vi "Modbus Status PC.vi"(0 "InterfaceData":T1 {"GenEast"."TotalFuel(L)" format="%.2f"; "GenEast"."FuelRate(L/H)" format="%.2f"; "GenEast"."ApparentPower(VA)" format="%.2f"; "GenEast"."BattVoltage(V)" format="%.2f"; "GenEast"."Freq(Hz)" format="%.2f"; "GenEast"."RunHours(hr)" format="%.2f"; "GenEast"."PowerFactor" format="%.2f"; "GenEast"."ReactivePower(VAR)" format="%.2f"; "GenEast"."ActivePower(W)" format="%.2f"; "GenWest"."TotalFuel(L)" format="%.2f"; "GenWest"."FuelRate(L/H)" format="%.2f"; "GenWest"."ApparentPower(VA)" format="%.2f"; "GenWest"."BattVoltage(V)" format="%.2f"; "GenWest"."Freq(Hz)" format="%.2f"; "GenWest"."RunHours(hr)" format="%.2f"; "GenWest"."PowerFactor" format="%.2f"; "GenWest"."ReactivePower(VAR)" format="%.2f"; "GenWest"."ActivePower(W)" format="%.2f"; "Converter Alarms 2" format="%016b"; "Converter Faults 2" format="%016b"; "Controller Faults" format="%016b"; "System Status" format="%016b"; "Converter Alarms 1" format="%016b"; "Converter Faults 1" format="%016b"; "Solar Faults" format="%016b"; "ES Rack 10 Alarms" format="%016b"; "ES Rack 9 Alarms" format="%016b"; "ES Rack 8 Alarms" format="%016b"; "ES Rack 7 Alarms" format="%016b"; "ES Rack 6 Alarms" format="%016b"; "ES Rack 5 Alarms" format="%016b"; "ES Rack 4 Alarms" format="%016b"; "ES Rack 3 Alarms" format="%016b"; "ES Rack 2 Alarms" format="%016b"; "ES Rack 1 Alarms" format="%016b"; "ES System Alarms" format="%016b"; "System Faults" format="%016b"; "ES Rack 10 Faults" format="%016b"; "ES Rack 9 Faults" format="%016b"; "ES Rack 8 Faults" format="%016b"; "ES Rack 7  Faults" format="%016b"; "ES Rack 6 Faults" format="%016b"; "ES Rack 5 Faults" format="%016b"; "ES Rack 4 Faults" format="%016b"; "ES Rack 3 Faults" format="%016b"; "ES Rack 2 Faults" format="%016b"; "ES Rack 1 Faults" format="%016b"; "ES System Faults" format="%016b"}, 5 "PC Data In":T4 {"Alarms 2" format="%016b"; "Faults 2" format="%016b"; "Alarms 1" format="%016b"; "Faults 1" format="%016b"; "Contactor FB" format="%.0b"; "DC Voltage SP" format="%2.1f"; "Clear Faults SP" format="%.0b"; "Neutral Current" format="%2.1f"; "AC Current - L2" format="%2.1f"; "AC Voltage - L2" format="%2.1f"; "Temperature" format="%2.1f"; "DC Voltage" format="%2.1f"; "AC Current SP" format="%2.1f"; "AC Voltage SP" format="%2.1f"; "Frequency SP" format="%2.1f"; "AC Frequency" format="%2.1f"; "AC Current - L1" format="%2.1f"; "AC Voltage- L1" format="%2.1f"}, 9 "FPGA Data In":T3 {"SSG Active Current" format="%2.1f"; "PV Reactive Power (L1)" format="%2.1f"; "PV Reactive Power (L2)" format="%2.1f"; "PV Total Reactive Power" format="%2.1f"; "Gen Reactive Power (L1)" format="%2.1f"; "Gen Reactive Power (L2)" format="%2.1f"; "Gen Total Reactive Power" format="%2.1f"; "SSG Reactive Power (L1)" format="%2.1f"; "SSG Reactive Power (L2)" format="%2.1f"; "SSG Total Reactive Power" format="%2.1f"; "PV Total Current" format="%2.1f"; "PV Total Voltage" format="%2.1f"; "PV Active Power (L1)" format="%2.1f"; "PV Active Power (L2)" format="%2.1f"; "PV App Power (L1)" format="%2.1f"; "PV App Power (L2)" format="%2.1f"; "PV Total Active Power" format="%2.1f"; "PV Total App Power" format="%2.1f"; "PV Arms (L1)" format="%2.1f"; "PV Arms (L2)" format="%2.1f"; "PV Vrms (L1)" format="%2.1f"; "PV Vrms (L2)" format="%2.1f"; "Gen Total Current" format="%2.1f"; "SSG Total Current" format="%2.1f"; "Gen Total Voltage" format="%2.1f"; "SSG Total Voltage" format="%2.1f"; "Gen Active Power (L1)" format="%2.1f"; "Gen Active Power (L2)" format="%2.1f"; "SSG Active Power (L1)" format="%2.1f"; "SSG Active Power (L2)" format="%2.1f"; "Gen App Power (L1)" format="%2.1f"; "Gen App Power (L2)" format="%2.1f"; "SSG App Power (L1)" format="%2.1f"; "SSG App Power (L2)" format="%2.1f"; "Gen Total Active Power" format="%2.1f"; "Gen Total App Power" format="%2.1f"; "Gen Arms (L1)" format="%2.1f"; "Gen Arms (L2)" format="%2.1f"; "Gen Vrms (L1)" format="%2.1f"; "Gen Vrms (L2)" format="%2.1f"; "SSG Total Active Power" format="%2.1f"; "SSG Total App Power" format="%2.1f"; "SSG Arms (L1)" format="%2.1f"; "SSG Arms (L2)" format="%2.1f"; "SSG Vrms (L1)" format="%2.1f"; "SSG Vrms (L2)" format="%2.1f"}, 11 "Error In":errorcluster) -> (4 "InterfaceData":T1 {"GenEast"."TotalFuel(L)" format="%.2f"; "GenEast"."FuelRate(L/H)" format="%.2f"; "GenEast"."ApparentPower(VA)" format="%.2f"; "GenEast"."BattVoltage(V)" format="%.2f"; "GenEast"."Freq(Hz)" format="%.2f"; "GenEast"."RunHours(hr)" format="%.2f"; "GenEast"."PowerFactor" format="%.2f"; "GenEast"."ReactivePower(VAR)" format="%.2f"; "GenEast"."ActivePower(W)" format="%.2f"; "GenWest"."TotalFuel(L)" format="%.2f"; "GenWest"."FuelRate(L/H)" format="%.2f"; "GenWest"."ApparentPower(VA)" format="%.2f"; "GenWest"."BattVoltage(V)" format="%.2f"; "GenWest"."Freq(Hz)" format="%.2f"; "GenWest"."RunHours(hr)" format="%.2f"; "GenWest"."PowerFactor" format="%.2f"; "GenWest"."ReactivePower(VAR)" format="%.2f"; "GenWest"."ActivePower(W)" format="%.2f"; "Converter Alarms 2" format="%016b"; "Converter Faults 2" format="%016b"; "Controller Faults" format="%016b"; "System Status" format="%016b"; "Converter Alarms 1" format="%016b"; "Converter Faults 1" format="%016b"; "Solar Faults" format="%016b"; "ES Rack 10 Alarms" format="%016b"; "ES Rack 9 Alarms" format="%016b"; "ES Rack 8 Alarms" format="%016b"; "ES Rack 7 Alarms" format="%016b"; "ES Rack 6 Alarms" format="%016b"; "ES Rack 5 Alarms" format="%016b"; "ES Rack 4 Alarms" format="%016b"; "ES Rack 3 Alarms" format="%016b"; "ES Rack 2 Alarms" format="%016b"; "ES Rack 1 Alarms" format="%016b"; "ES System Alarms" format="%016b"; "System Faults" format="%016b"; "ES Rack 10 Faults" format="%016b"; "ES Rack 9 Faults" format="%016b"; "ES Rack 8 Faults" format="%016b"; "ES Rack 7  Faults" format="%016b"; "ES Rack 6 Faults" format="%016b"; "ES Rack 5 Faults" format="%016b"; "ES Rack 4 Faults" format="%016b"; "ES Rack 3 Faults" format="%016b"; "ES Rack 2 Faults" format="%016b"; "ES Rack 1 Faults" format="%016b"; "ES System Faults" format="%016b"}, 15 "Error Out":errorcluster)   [LabVIEW 2014]
uses:
  Controls/PC Data.ctl
  Controls/MicroZed Config Op Mode.ctl
  Controls/FPGA Data.ctl
  Controls/Interface Data.ctl
  Controls/Gen Data.ctl
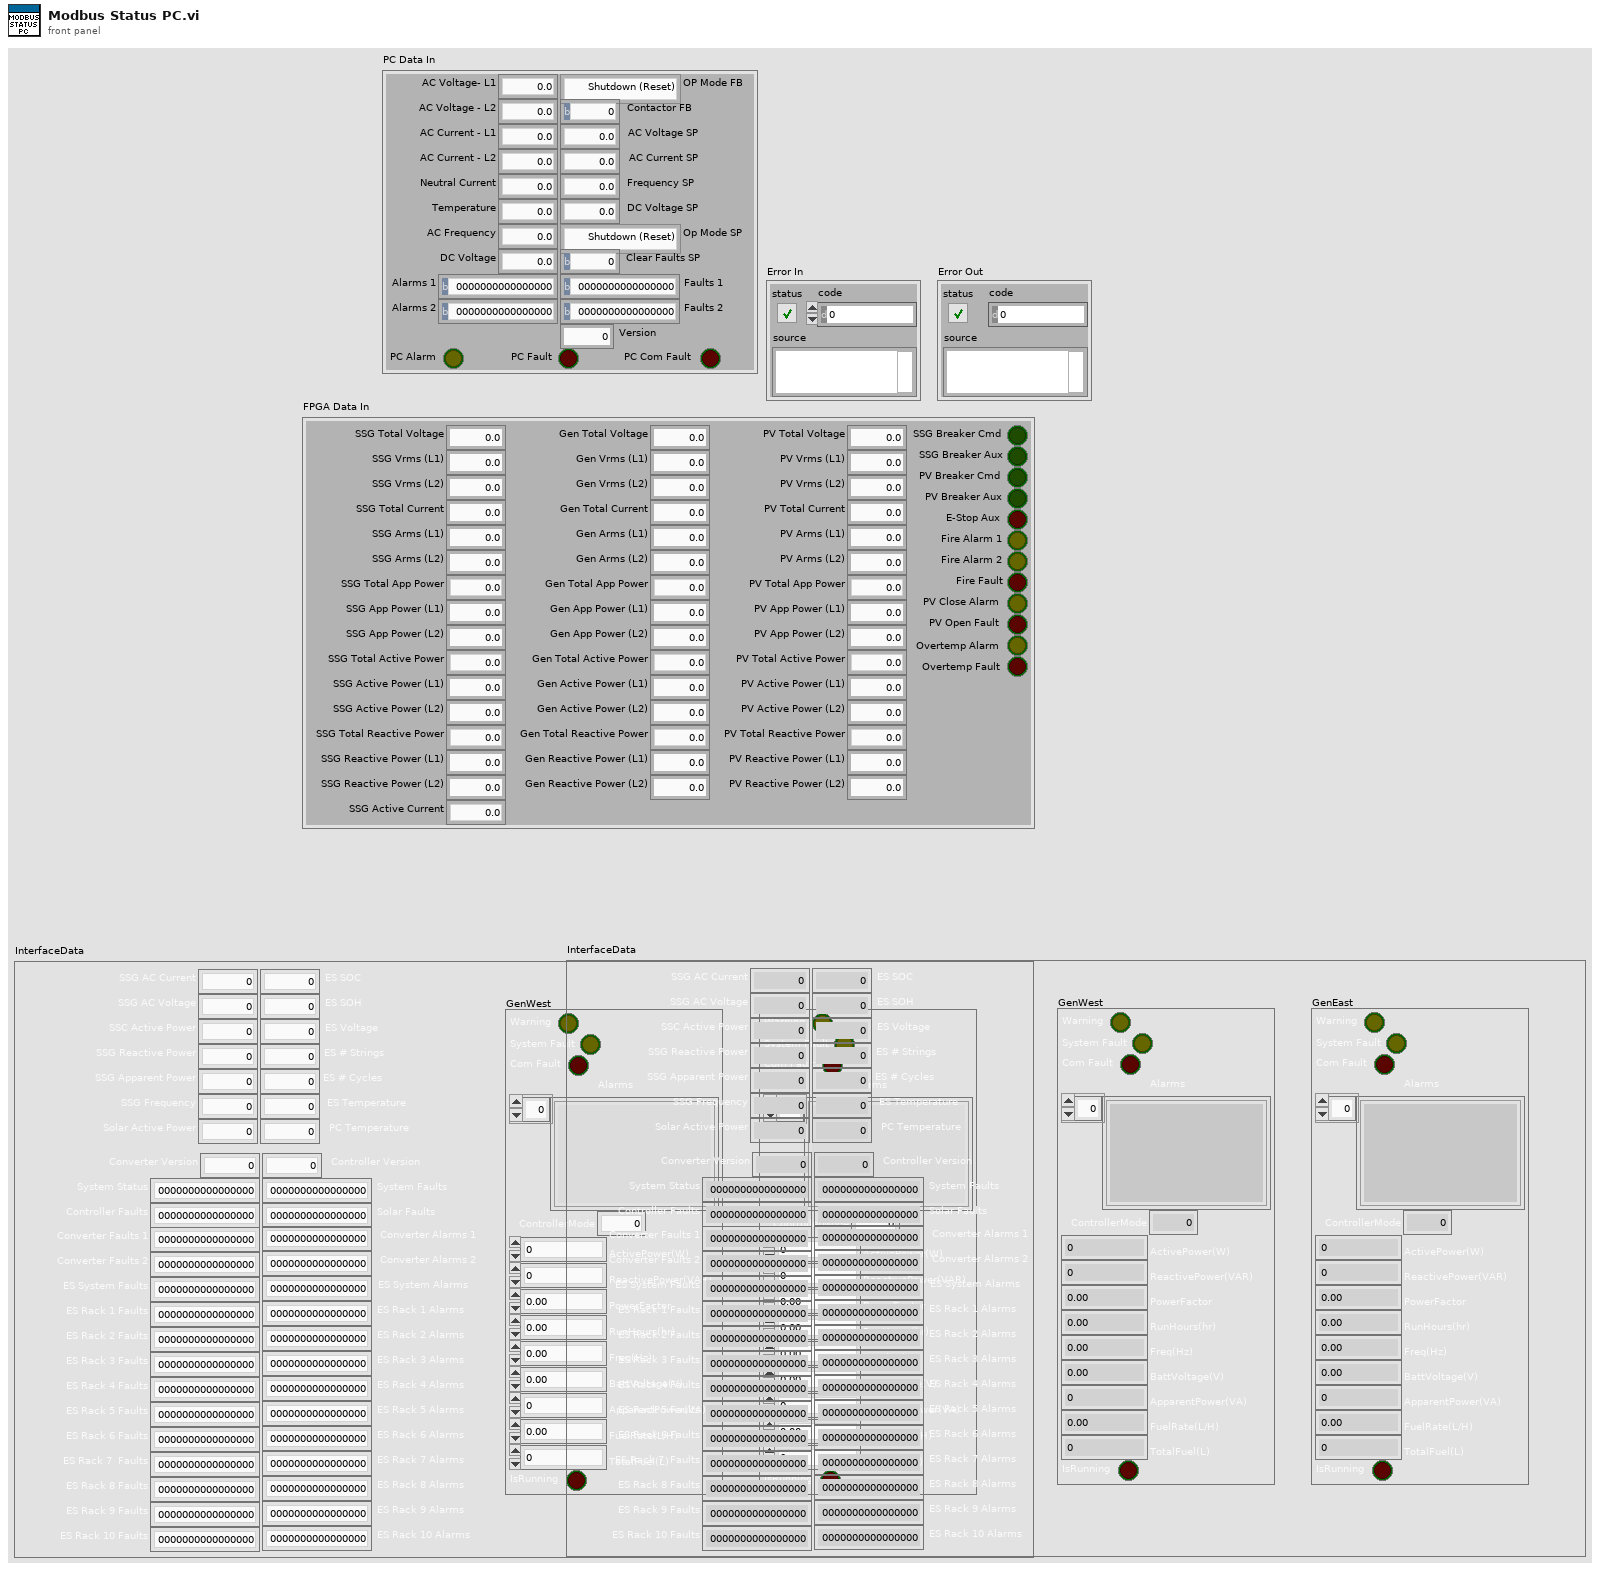
[diagram p1: front panel]
types:
  T1 = typedef "Interface Data.ctl" = cluster{"SSG AC Current":i16, "SSG AC Voltage":i16, "SSC Active Power":i16, "SSG Reactive Power":i16, "SSG Apparent Power":i16, "SSG Frequency":i16, "ES SOC":i16, "ES SOH":i16, "ES Voltage":i16, "ES # Strings":i16, "ES # Cycles":i16, "ES Temperature":i16, "PC Temperature":i16, "Solar Active Power":i16, "Converter Version":i16, "Controller Version":i16, "System Status":i16, "System Faults":i16, "Controller Faults":i16, "ES System Faults":i16, "ES System Alarms":i16, "Converter Faults 1":i16, "Converter Faults 2":i16, "Converter Alarms 1":i16, "Converter Alarms 2":i16, "Solar Faults":i16, "ES Rack 1 Faults":i16, "ES Rack 2 Faults":i16, "ES Rack 3 Faults":i16, "ES Rack 4 Faults":i16, "ES Rack 5 Faults":i16, "ES Rack 6 Faults":i16, "ES Rack 7  Faults":i16, "ES Rack 8 Faults":i16, "ES Rack 9 Faults":i16, "ES Rack 10 Faults":i16, "ES Rack 1 Alarms":i16, "ES Rack 2 Alarms":i16, "ES Rack 3 Alarms":i16, "ES Rack 4 Alarms":i16, "ES Rack 5 Alarms":i16, "ES Rack 6 Alarms":i16, "ES Rack 7 Alarms":i16, "ES Rack 8 Alarms":i16, "ES Rack 9 Alarms":i16, "ES Rack 10 Alarms":i16, "GenWest":T2, "GenEast":T2}
  T2 = typedef "Gen Data.ctl" = cluster{"Warning":bool, "System Fault":bool, "Com Fault":bool, "Alarms":string[], "ControllerMode":u16, "ActivePower(W)":i32, "ReactivePower(VAR)":i32, "PowerFactor":dbl, "RunHours(hr)":dbl, "Freq(Hz)":dbl, "BattVoltage(V)":dbl, "ApparentPower(VA)":i32, "FuelRate(L/H)":dbl, "TotalFuel(L)":u32, "IsRunning":bool}
  T3 = typedef "FPGA Data.ctl" = cluster{"Gen Total Voltage":dbl, "Gen Vrms (L1)":dbl, "Gen Vrms (L2)":dbl, "Gen Total Current":dbl, "Gen Arms (L1)":dbl, "Gen Arms (L2)":dbl, "Gen Total App Power":dbl, "Gen App Power (L1)":dbl, "Gen App Power (L2)":dbl, "Gen Total Active Power":dbl, "Gen Active Power (L1)":dbl, "Gen Active Power (L2)":dbl, "Gen Total Reactive Power":dbl, "Gen Reactive Power (L1)":dbl, "Gen Reactive Power (L2)":dbl, "SSG Total Voltage":dbl, "SSG Vrms (L1)":dbl, "SSG Vrms (L2)":dbl, "SSG Total Current":dbl, "SSG Arms (L1)":dbl, "SSG Arms (L2)":dbl, "SSG Total App Power":dbl, "SSG App Power (L1)":dbl, "SSG App Power (L2)":dbl, "SSG Total Active Power":dbl, "SSG Active Power (L1)":dbl, "SSG Active Power (L2)":dbl, "SSG Total Reactive Power":dbl, "SSG Reactive Power (L1)":dbl, "SSG Reactive Power (L2)":dbl, "PV Total Voltage":dbl, "PV Vrms (L1)":dbl, "PV Vrms (L2)":dbl, "PV Total Current":dbl, "PV Arms (L1)":dbl, "PV Arms (L2)":dbl, "PV Total App Power":dbl, "PV App Power (L1)":dbl, "PV App Power (L2)":dbl, "PV Total Active Power":dbl, "PV Active Power (L1)":dbl, "PV Active Power (L2)":dbl, "PV Total Reactive Power":dbl, "PV Reactive Power (L1)":dbl, "PV Reactive Power (L2)":dbl, "SSG Breaker Cmd":bool, "SSG Breaker Aux":bool, "PV Breaker Cmd":bool, "PV Breaker Aux":bool, "E-Stop Aux":bool, "Fire Alarm 1":bool, "Fire Alarm 2":bool, "Fire Fault":bool, "PV Close Alarm":bool, "SSG Active Current":dbl, "Overtemp Alarm":bool, "Overtemp Fault":bool, "PV Open Fault":bool}
  T4 = typedef "PC Data.ctl" = cluster{"AC Voltage- L1":dbl, "AC Voltage - L2":dbl, "AC Current - L1":dbl, "AC Current - L2":dbl, "Neutral Current":dbl, "Temperature":dbl, "AC Frequency":dbl, "DC Voltage":dbl, "AC Voltage SP":dbl, "AC Current SP":dbl, "Frequency SP":dbl, "Op Mode SP":T5, "Clear Faults SP":u16, "PC Com Fault":bool, "PC Fault":bool, "DC Voltage SP":dbl, "OP Mode FB":T5, "Contactor FB":u16, "Faults 1":u16, "Alarms 1":u16, "Faults 2":u16, "Alarms 2":u16, "PC Alarm":bool, "Version":u16}
  T5 = typedef "MicroZed Config Op Mode.ctl" = enum16{"Shutdown (Reset)", "Startup", "Idle", "Voltage Mode", "Current Mode", "Fault", "OL Voltage (Debug)", "No Data"}
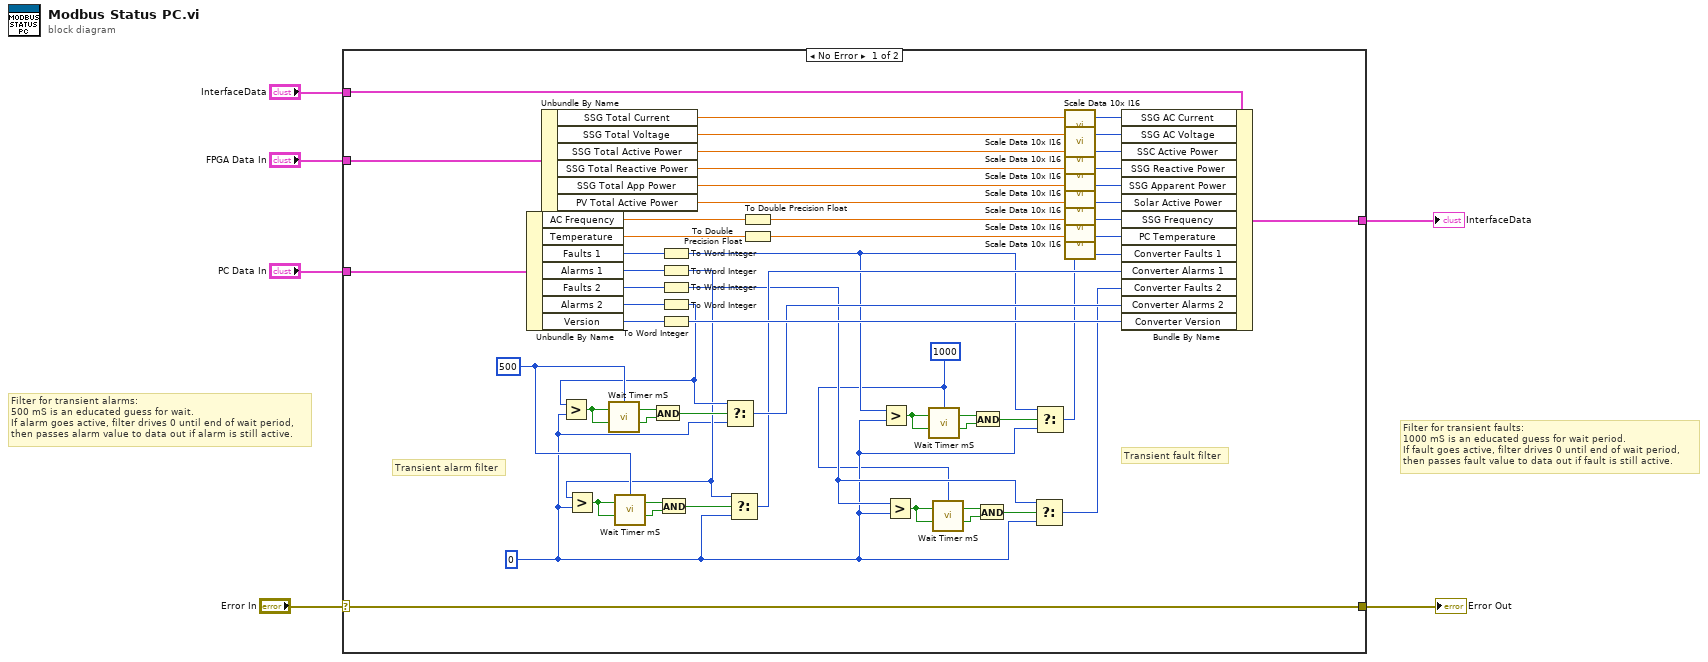
[diagram p0: block diagram]
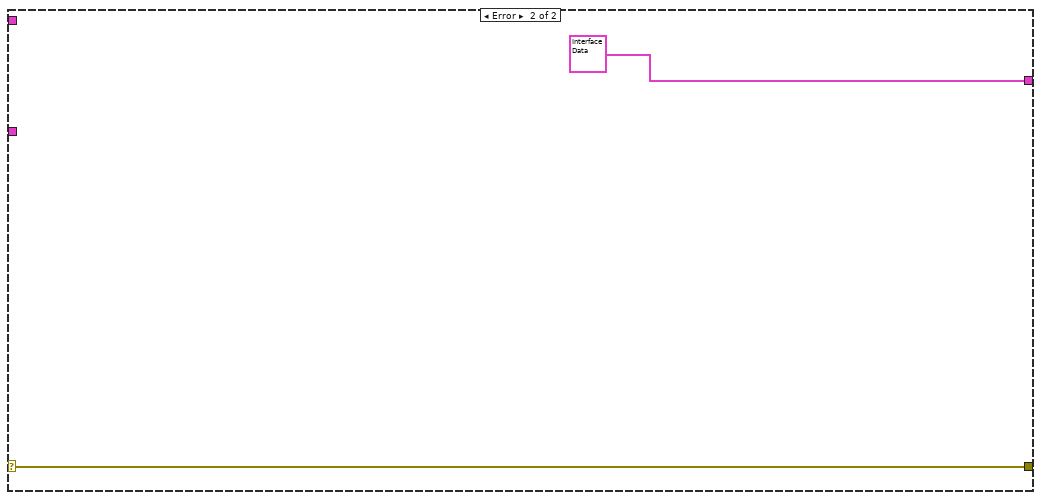
[diagram p2: hidden frame]
diagram:
  # "Filter for transient faults:\n1000 mS is an educated guess for wait period.\nIf fault goes active, filter drives 0 until end of wait period,\nthen passes fault value to data out if fault is still active."
  # "Filter for transient alarms:\n500 mS is an educated guess for wait.\nIf alarm goes active, filter drives 0 until end of wait period,\nthen passes alarm value to data out if alarm is still active."
  n1 = case shown="No Error" "Error In" {
    selector: "Error In" -> [w58 w60]
    tunnel: [w58 w60] -> w5
    tunnel: "InterfaceData" -> [w57 _]
    tunnel: [w56 T1 {"SSG AC Current"=0, "SSG AC Voltage"=0, "SSC Active Power"=0, "SSG Reactive Power"=0, "SSG Apparent Power"=0, "SSG Frequency"=0, "ES SOC"=0, "ES SOH"=0, "ES Voltage"=0, "ES # Strings"=0, "ES # Cycles"=0, "ES Temperature"=0, "PC Temperature"=0, "Solar Active Power"=0, "Converter Version"=0, "Controller Version"=0, "System Status"=0, "System Faults"=0, "Controller Faults"=0, "ES System Faults"=0, "ES System Alarms"=0, "Converter Faults 1"=0, "Converter Faults 2"=0, "Converter Alarms 1"=0, "Converter Alarms 2"=0, "Solar Faults"=0, "ES Rack 1 Faults"=0, "ES Rack 2 Faults"=0, "ES Rack 3 Faults"=0, "ES Rack 4 Faults"=0, "ES Rack 5 Faults"=0, "ES Rack 6 Faults"=0, "ES Rack 7  Faults"=0, "ES Rack 8 Faults"=0, "ES Rack 9 Faults"=0, "ES Rack 10 Faults"=0, "ES Rack 1 Alarms"=0, "ES Rack 2 Alarms"=0, "ES Rack 3 Alarms"=0, "ES Rack 4 Alarms"=0, "ES Rack 5 Alarms"=0, "ES Rack 6 Alarms"=0, "ES Rack 7 Alarms"=0, "ES Rack 8 Alarms"=0, "ES Rack 9 Alarms"=0, "ES Rack 10 Alarms"=0, "GenWest"={"Warning"=FALSE, "System Fault"=FALSE, "Com Fault"=FALSE, "Alarms"=[], "ControllerMode"=0, "ActivePower(W)"=0, "ReactivePower(VAR)"=0, "PowerFactor"=0.0, "RunHours(hr)"=0.0, "Freq(Hz)"=0.0, "BattVoltage(V)"=0.0, "ApparentPower(VA)"=0, "FuelRate(L/H)"=0.0, "TotalFuel(L)"=0, "IsRunning"=FALSE}, "GenEast"={"Warning"=FALSE, "System Fault"=FALSE, "Com Fault"=FALSE, "Alarms"=[], "ControllerMode"=0, "ActivePower(W)"=0, "ReactivePower(VAR)"=0, "PowerFactor"=0.0, "RunHours(hr)"=0.0, "Freq(Hz)"=0.0, "BattVoltage(V)"=0.0, "ApparentPower(VA)"=0, "FuelRate(L/H)"=0.0, "TotalFuel(L)"=0, "IsRunning"=FALSE}} ("Modbus Status Interface Data In")] -> w3
    tunnel: "FPGA Data In" -> [w55 _]
    tunnel: "PC Data In" -> [w54 _]
    frame No Error {
      w7 = u32 1000 ("Timer")
      w8 = i16 0 ("y")
      w23 = u32 500 ("Timer")
      # "Transient alarm filter"
      # "Transient fault filter"
      n2 = Unbundle By Name(w54) -> ("AC Frequency"=w45:dbl, "Temperature"=w44:dbl, "Faults 1"=w35:u16, "Alarms 1"=w34:u16, "Faults 2"=w33:u16, "Alarms 2"=w32:u16, "Version"=w31:u16)
      n3 = Unbundle By Name(w55) -> ("SSG Total Current"=w51:dbl, "SSG Total Voltage"=w53:dbl, "SSG Total Active Power"=w49:dbl, "SSG Total Reactive Power"=w48:dbl, "SSG Total App Power"=w47:dbl, "PV Total Active Power"=w46:dbl)
      n4 = To Word Integer(number=w35) -> (16bit integer=w12:i16)
      n5 = To Word Integer(number=w34) -> (16bit integer=w20:i16)
      n6 = Greater?(x=w20, y=w8) -> (0:w25:bool)
      n7 = call "Wait Timer mS.vi"("Boolean In"=w25, "Timer"=w23) -> ("Boolean Out"=w24:bool)  [unwired: 3 in]
      n8 = And(x=w24, y=w25) -> (x .and. y?=w26:bool)
      n9 = To Word Integer(number=w33) -> (16bit integer=w10:i16)
      n10 = To Word Integer(number=w32) -> (16bit integer=w21:i16)
      n11 = Greater?(x=w21, y=w8) -> (0:w28:bool)
      n12 = call "Wait Timer mS.vi"("Boolean In"=w28, "Timer"=w23) -> ("Boolean Out"=w29:bool)  [unwired: 3 in]
      n13 = And(x=w29, y=w28) -> (x .and. y?=w27:bool)
      n14 = To Word Integer(number=w31) -> (16bit integer=w30:i16)
      n15 = Select(t=w21, s=w27, f=w8) -> (s? t:f=w22:i16)
      n16 = Select(t=w20, s=w26, f=w8) -> (s? t:f=w19:i16)
      n17 = To Double Precision Float(number=w45) -> (double precision float=w42:dbl)
      n18 = To Double Precision Float(number=w44) -> (double precision float=w43:dbl)
      n19 = Greater?(x=w12, y=w8) -> (0:w14:bool)
      n20 = Greater?(x=w10, y=w8) -> (0:w17:bool)
      n21 = call "Wait Timer mS.vi"("Boolean In"=w14, "Timer"=w7) -> ("Boolean Out"=w13:bool)  [unwired: 3 in]
      n22 = call "Wait Timer mS.vi"("Boolean In"=w17, "Timer"=w7) -> ("Boolean Out"=w18:bool)  [unwired: 3 in]
      n23 = And(x=w13, y=w14) -> (x .and. y?=w15:bool)
      n24 = And(x=w18, y=w17) -> (x .and. y?=w16:bool)
      n25 = Select(t=w10, s=w16, f=w8) -> (s? t:f=w9:i16)
      n26 = Select(t=w12, s=w15, f=w8) -> (s? t:f=w11:i16)
      n27 = call "Scale Data 10x I16.vi"("Data In"=w51) -> ("16bit integer"=w50:i16)  [unwired: 2 in]
      n28 = call "Scale Data 10x I16.vi"("Data In"=w53) -> ("16bit integer"=w52:i16)  [unwired: 2 in]
      n29 = call "Scale Data 10x I16.vi"("Data In"=w49) -> ("16bit integer"=w41:i16)  [unwired: 2 in]
      n30 = call "Scale Data 10x I16.vi"("Data In"=w48) -> ("16bit integer"=w40:i16)  [unwired: 2 in]
      n31 = call "Scale Data 10x I16.vi"("Data In"=w47) -> ("16bit integer"=w39:i16)  [unwired: 2 in]
      n32 = call "Scale Data 10x I16.vi"("Data In"=w46) -> ("16bit integer"=w38:i16)  [unwired: 2 in]
      n33 = call "Scale Data 10x I16.vi"("Data In"=w42) -> ("16bit integer"=w37:i16)  [unwired: 2 in]
      n34 = call "Scale Data 10x I16.vi"("Data In"=w43) -> ("16bit integer"=w36:i16)  [unwired: 2 in]
      n35 = Bundle By Name(cluster=w57, "SSG AC Current"=w50, "SSG AC Voltage"=w52, "SSC Active Power"=w41, "SSG Reactive Power"=w40, "SSG Apparent Power"=w39, "Solar Active Power"=w38, "SSG Frequency"=w37, "PC Temperature"=w36, "Converter Faults 1"=w11, "Converter Alarms 1"=w19, "Converter Faults 2"=w9, "Converter Alarms 2"=w22, "Converter Version"=w30) -> (w56:T1)
    }
    frame Error {
    }
  }
  "Error Out" <- w5
  "InterfaceData" <- w3
